vi "Read Attributes.vi"(11 "Case-Controller Msg":refnum<class "Case-Controller Msg.lvclass">) -> (2 "Payload":cluster{"Controller Case":string})   [LabVIEW 2025, in "UserConsole.lvlib" / "Case-Controller Msg.lvclass"]
uses:
  Case-Controller Msg.lvclass
  Case-Controller Msg.lvclass/Case-Controller Msg.ctl
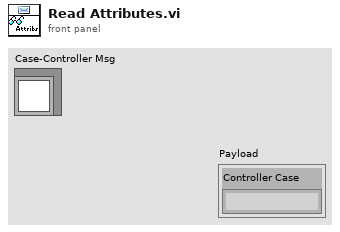
[diagram p1: front panel]
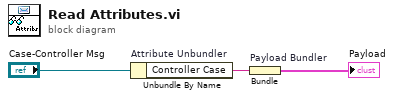
[diagram p0: block diagram]
diagram:
  n1 = Unbundle By Name "Attribute Unbundler"("Case-Controller Msg") -> ("Controller Case"=w1:string)
  n2 = Bundle "Payload Bundler"("Controller Case"=w1) -> (→"Payload":cluster{"Controller Case":string})  [unwired: 1 in]
